vi "05_2.vi"() -> ()   [LabVIEW 2018]
panel:
  out "Array":i32[](array[numeric])
  in  "String":string
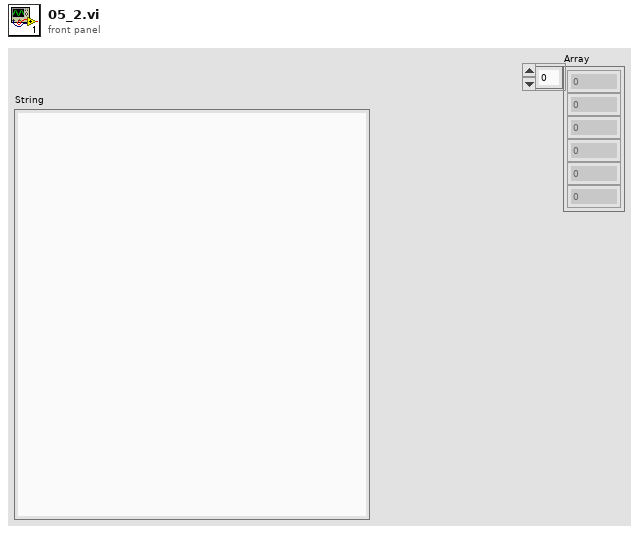
[diagram p1: front panel]
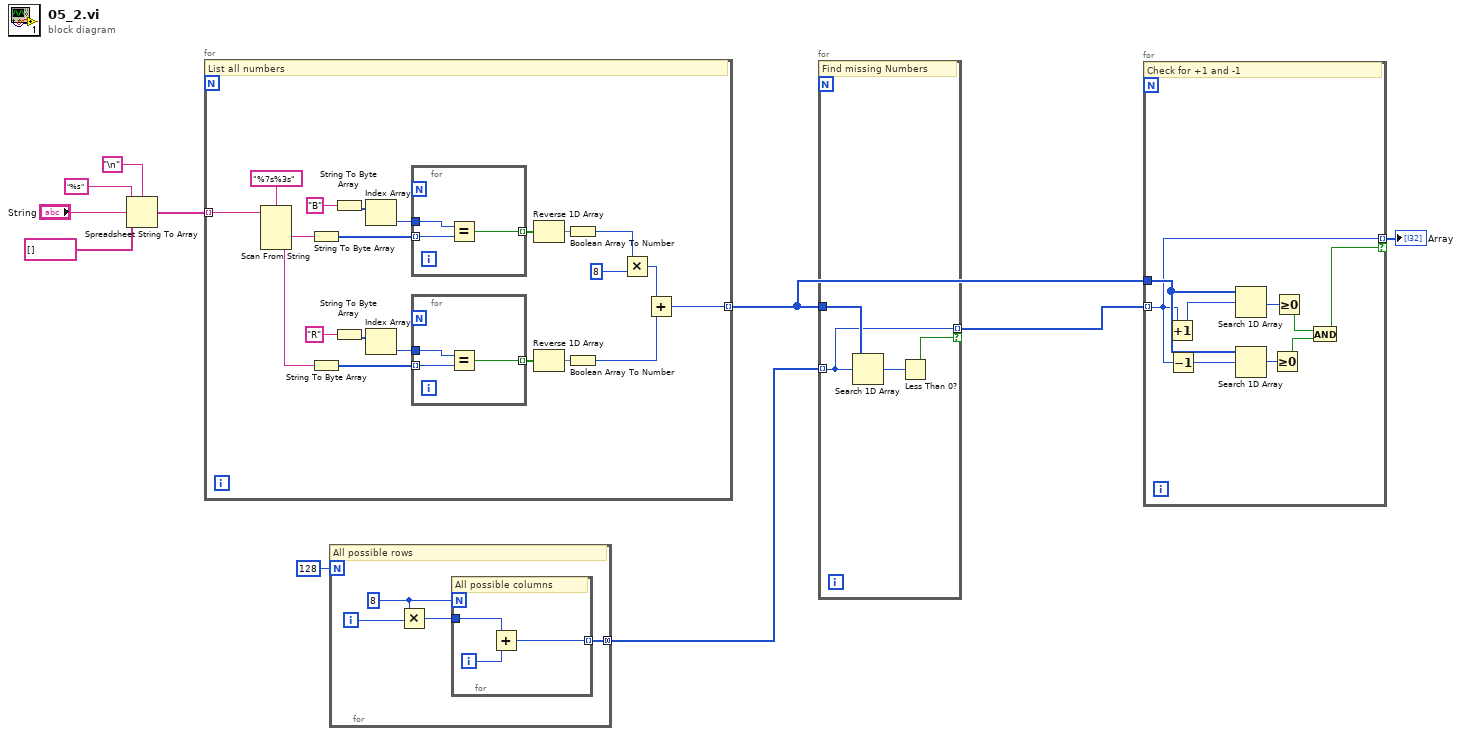
[diagram p0: block diagram]
diagram:
  n1 = Spreadsheet String To Array(delimiter (Tab)="\n", format string="%s", spreadsheet string="String", array type (2D Dbl)=string[] []) -> (array=w6:string[])
  n2 = for {
    tunnel: w6 -> [w31] mode=indexing
    tunnel: [w13] -> w2 mode=indexing
    # "List all numbers"
    n3 = Scan From String(format string="%7s%3s", input string=w31) -> (output 1=w29:string, output 2=w18:string)  [unwired: 4 in, 3 out]
    n4 = String To Byte Array(string=w29) -> (unsigned byte array=w28:u8[])
    n5 = String To Byte Array(string=w18) -> (unsigned byte array=w19:u8[])
    n6 = String To Byte Array(string="B") -> (unsigned byte array=w25:u8[])
    n7 = String To Byte Array(string="R") -> (unsigned byte array=w22:u8[])
    n8 = Index Array(array=w25) -> (element=w24:u8)  [unwired: 1 in]
    n9 = Index Array(array=w22) -> (element=w23:u8)  [unwired: 1 in]
    n10 = for {
      tunnel: w28 -> [w37] mode=indexing
      tunnel: [w36] -> w27 mode=indexing
      tunnel: w24 -> [w35]
      n11 = Equal?(x=w35, y=w37) -> (x = y?=w36:bool)
    }
    n12 = for {
      tunnel: w19 -> [w34] mode=indexing
      tunnel: [w33] -> w20 mode=indexing
      tunnel: w23 -> [w32]
      n13 = Equal?(x=w32, y=w34) -> (x = y?=w33:bool)
    }
    n14 = Reverse 1D Array(array=w27) -> (reversed array=w17:bool[])
    n15 = Reverse 1D Array(array=w20) -> (reversed array=w16:bool[])
    n16 = Boolean Array To Number(Boolean array=w17) -> (number=w11:u32)
    n17 = Boolean Array To Number(Boolean array=w16) -> (number=w12:u32)
    n18 = Multiply(x=w11, y=8) -> (x*y=w14:u32)
    n19 = Add(x=w14, y=w12) -> (x+y=w13:u32)
  }
  n20 = for {
    N: 128 -> [_]
    tunnel: [w38] -> w4 mode=concatenating
    i -> [w40]
    w41 = 8
    # "All possible rows"
    n21 = Multiply(x=w41, y=w40) -> (x*y=w39:i32)
    n22 = for {
      N: w41 -> [_]
      tunnel: w39 -> [w43]
      tunnel: [w42] -> w38 mode=indexing
      i -> [w44]
      # "All possible columns"
      n23 = Add(x=w43, y=w44) -> (x+y=w42:i32)
    }
  }
  n24 = for {
    tunnel: w2 -> [w48]
    tunnel: w4 -> [w46] mode=indexing
    tunnel: [w46] -> w3 mode=indexing if=w45
    # "Find missing Numbers"
    n25 = Search 1D Array(1D array=w48, element=w46) -> (index of element=w47:i32)  [unwired: 1 in]
    n26 = Less Than 0?(x=w47) -> (x < 0?=w45:bool)
  }
  n27 = for {
    tunnel: w3 -> [w50] mode=indexing
    tunnel: w2 -> [w56]
    tunnel: [w50] -> w1 mode=indexing if=w49
    # "Check for +1 and -1"
    n28 = Increment(x=w50) -> (x+1=w57:i32)
    n29 = Decrement(x=w50) -> (x-1=w55:i32)
    n30 = Search 1D Array(1D array=w56, element=w57) -> (index of element=w53:i32)  [unwired: 1 in]
    n31 = Search 1D Array(1D array=w56, element=w55) -> (index of element=w54:i32)  [unwired: 1 in]
    n32 = Greater Or Equal To 0?(x=w54) -> (x >= 0?=w52:bool)
    n33 = Greater Or Equal To 0?(x=w53) -> (x >= 0?=w51:bool)
    n34 = And(x=w51, y=w52) -> (x .and. y?=w49:bool)
  }
  "Array" <- w1
